vi "Main Tclk.vi"() -> ()   [LabVIEW 2018] (continued)
                  frame False {
                    n1784 = local read "AlnX array tiled"() -> (w6252:sgl[][][])
                    n1785 = local read "AlnY array tiled"() -> (w6253:sgl[][][])
                    n1786 = local read "Auto Focus"() -> (w6257:bool)
                    n1787 = local read "Auto Stig"() -> (w6258:bool)
                    n1788 = Empty Array?(array=w6252) -> (empty?=w6251:bool)
                    n1789 = Empty Array?(array=w6253) -> (empty?=w6250:bool)
                    n1790 = local write "Aln Options"(enum16{"Defaut", "Aln X", "Aln Y"}."Defaut" ("Stig Options")) -> ()
                    n1791 = Not(x=w6257) -> (.not. x?=w6259:bool)
                    n1792 = Not(x=w6258) -> (.not. x?=w6260:bool)
                    n1793 = And(x=w6251, y=w6250) -> (x .and. y?=w6255:bool)
                    n1794 = Compound Arithmetic op=AND(w6255, w6259, w6260) -> (w6256:bool)
                    n1795 = case shown="False" w6255 {
                      frame False {
                        n1796 = property on="Auto Align" class="Bool (strict)"("DisabledEnum"=T44."Disabled and Grayed Out" ("Disabled")) -> ()  [unwired: 2 in, 2 out]
                      }
                      frame True {
                      }
                    }
                    n1797 = case shown="True" w6256 {
                      frame False {
                      }
                      frame True {
                        w6261 = T44."Enabled" ("Disabled")
                        n1798 = property on="Auto Focus" class="Bool (strict)"("DisabledEnum"=w6261) -> ()  [unwired: 2 in, 2 out]
                        n1799 = property on="Auto Stig" class="Bool (strict)"("DisabledEnum"=w6261) -> ()  [unwired: 2 in, 2 out]
                      }
                    }
                  }
                  frame True {
                    w6265 = T44."Disabled and Grayed Out" ("Disabled")
                    n1800 = local read "SEM Scan Parameters"() -> (w6269:T26)
                    n1801 = local read "AA Count"() -> (w6264:u8)
                    n1802 = local read "Aln Options"() -> (w6273:enum16{"Defaut", "Aln X", "Aln Y"})
                    n1803 = Increment(x=w6264) -> (x+1=w6270:u8)
                    n1804 = Equal To 0?(x=w6264) -> (x = 0?=w6263:bool)
                    n1805 = local write "AA Count"(w6270) -> ()
                    n1806 = Unbundle By Name(w6269) -> ("Y tiles"=w6268:u8, "X tiles"=w6267:u8)
                    n1807 = Equal?(x=w6273, y=enum16{"Defaut", "Aln X", "Aln Y"}."Defaut" ("Aln Options")) -> (x = y?=w6271:bool)
                    n1808 = property on="Auto Focus" class="Bool (strict)"("DisabledEnum"=w6265) -> ()  [unwired: 2 in, 2 out]
                    n1809 = And(x=w6263, y=w6271) -> (x .and. y?=w6272:bool)
                    n1810 = case shown="True" w6272 {
                      tunnel: w6268 -> [_ w6277]
                      tunnel: w6267 -> [_ w6276]
                      frame False {
                      }
                      frame True {
                        n1811 = Initialize Array(FALSE ("ASX Success"), w6277, w6276) -> (w6280:bool[][])
                        n1812 = Initialize Array(u8 0 ("Skip Steps"), w6277, w6276) -> (w6275:u8[][])
                        n1813 = local write "AAX Success tiled"(w6280) -> ()
                        n1814 = local write "AAY Success tiled"(w6280) -> ()
                        n1815 = local write "Skip Steps tiled"(w6275) -> ()
                        n1816 = local write "Aln Options"(enum16{"Defaut", "Aln X", "Aln Y"}."Aln X" ("Stig Options")) -> ()
                        n1817 = local write "Image Tabs"(T37."Auto Focus / Stig / Align" ("Image Tabs")) -> ()
                      }
                    }
                    n1818 = property on="Auto Stig" class="Bool (strict)"("DisabledEnum"=w6265) -> ()  [unwired: 2 in, 2 out]
                  }
                }
              }
              frame #16 {
                n1819 = local read "SEM Scan Parameters"() -> (w6319:T26)
                n1820 = local read "FIB slice #"() -> (w6329:u32)
                n1821 = local read "Machine Type"() -> (w6316:u8)
                n1822 = shared-variable "My Computer\\Zeiss Library.lvlib\\FIB Slice #"(w6329) -> ()  [unwired: 1 in, 1 out]
                n1823 = Equal To 0?(x=w6329) -> (x = 0?=w6352:bool)
                n1824 = Or(x=w6352, y="Reset Focus") -> (x .or. y?=w6321:bool)
                n1825 = local read "Milling para"() -> (w6345:T35)
                n1826 = local read "FIB-SEM Angle"() -> (w6348:dbl)
                n1827 = case shown="False" w6321 {
                  tunnel: [w6358 w6365] -> w6325
                  tunnel: [w6357 w6364] -> w6324
                  tunnel: [w6356 w6363] -> w6326
                  tunnel: [w6355 w6362] -> w6323
                  tunnel: [w6354 w6361] -> w6322
                  tunnel: w6319 -> [w6353 w6360]
                  tunnel: w6316 -> [_ w6359]
                  frame False {
                    n1828 = Unbundle By Name(w6353) -> ("WD (mm)"=w6356:sgl[][], "X stig"=w6358:sgl[][], "Y stig"=w6357:sgl[][], "X aln"=w6355:sgl[][], "Y aln"=w6354:sgl[][])
                  }
                  frame True {
                    n1829 = stacked-sequence {
                      tunnel: [_ w6373] -> w6365
                      tunnel: [_ w6372] -> w6364
                      tunnel: [_ w6371] -> w6363
                      tunnel: [_ w6370] -> w6362
                      tunnel: [_ w6369] -> w6361
                      tunnel: w6360 -> [_ w6368]
                      tunnel: w6359 -> [_ w6367]
                      frame #0 {
                        n1830 = local read "SEM Options"() -> (→"Initial Options":T27)
                      }
                      frame #1 {
                        n1831 = case shown="2" w6367 {
                          tunnel: [w6381 w6460] -> w6373
                          tunnel: [w6380 w6459] -> w6372
                          tunnel: [w6379 w6461] -> w6371
                          tunnel: [w6378 w6458] -> w6370
                          tunnel: [w6377 w6457] -> w6369
                          tunnel: w6368 -> [w6374 _]
                          frame 0, Default {
                            n1832 = local read "Hardware Configuration"() -> (w6376:T25)
                            n1833 = Unbundle By Name(w6376) -> ("Eanable COM"=w6375:bool)
                            n1834 = case shown="True" w6375 {
                              tunnel: [w6385 w6395] -> w6381
                              tunnel: [w6384 w6394] -> w6380
                              tunnel: [w6386 w6400] -> w6379
                              tunnel: [w6383 w6393] -> w6378
                              tunnel: [w6382 w6392] -> w6377
                              tunnel: w6374 -> [w6387 _]
                              frame False {
                                n1835 = Unbundle By Name(w6387) -> ("WD (mm)"=w6386:sgl[][], "X stig"=w6385:sgl[][], "Y stig"=w6384:sgl[][], "X aln"=w6383:sgl[][], "Y aln"=w6382:sgl[][])
                              }
                              frame True {
                                w6414 = TRUE ("Initialization")
                                w6405 = 0 ("offset past token")
                                n1836 = local read "COM port"() -> (w6418:refnum<visa-resource-name>)
                                n1837 = call "Remcon32 command.vi"("Initialization"=w6414, "SEM command"="sti? " ("write buffer"), "COM port in"=w6418) -> ("error out"=w6408:errorcluster, "SEM reply"=w6415:string, "COM port out"=w6410:refnum<visa-resource-name>)  [unwired: 2 in, 4 out]
                                n1838 = while {
                                shift-right: [w6436] -> _
                                shift-left: w6405 -> [w6439]
                                tunnel: [w6437] -> w6421 mode=indexing
                                tunnel: w6415 -> [w6434]
                                stop <- w6435 stop-if-true
                                n1839 = Scan String For Tokens(8:w6439, 9:w6434) -> (1:w6437:string, 2:w6436:i32)  [unwired: 1 in, 5 out]
                                n1840 = Less?(x=w6436, y=0) -> (x < y?=w6435:bool)
                                }
                                n1841 = call "Remcon32 command.vi"("error in"=w6408, "SEM command"="aln? " ("write buffer"), "COM port in"=w6410) -> ("error out"=w6407:errorcluster, "SEM reply"=w6406:string, "COM port out"=w6409:refnum<visa-resource-name>)  [unwired: 2 in, 4 out]
                                n1842 = while {
                                shift-right: [w6427] -> _
                                shift-left: w6405 -> [w6430]
                                tunnel: [w6428] -> w6411 mode=indexing
                                tunnel: w6406 -> [w6425]
                                stop <- w6426 stop-if-true
                                n1843 = Scan String For Tokens(8:w6430, 9:w6425) -> (1:w6428:string, 2:w6427:i32)  [unwired: 1 in, 5 out]
                                n1844 = Less?(x=w6427, y=0) -> (x < y?=w6426:bool)
                                }
                                n1845 = for {
                                tunnel: w6421 -> [w6433] mode=indexing
                                tunnel: [w6432] -> w6420 mode=indexing
                                n1846 = Fract/Exp String To Number(string=w6433, default (0 dbl)=sgl 0.0 ("default (0 DBL)")) -> (number=w6432:sgl)  [unwired: 3 out]
                                }
                                n1847 = for {
                                tunnel: w6411 -> [w6424] mode=indexing
                                tunnel: [w6423] -> w6412 mode=indexing
                                n1848 = Fract/Exp String To Number(string=w6424, default (0 dbl)=sgl 0.0 ("default (0 DBL)")) -> (number=w6423:sgl)  [unwired: 3 out]
                                }
                                n1849 = call "Remcon32 command.vi"("Close session"=w6414, "error in"=w6407, "SEM command"="foc? " ("write buffer"), "COM port in"=w6409) -> ("SEM reply"=w6416:string)  [unwired: 1 in, 6 out]
                                n1850 = local read "WD Stig Aln tile offsets"() -> (w6403:T3)
                                n1851 = Fract/Exp String To Number(string=w6416, default (0 dbl)=sgl 0.0 ("default (0 DBL)")) -> (number=w6401:sgl)  [unwired: 3 out]
                                n1852 = Index Array(array=w6420) -> (element #1=w6391:sgl, element #2=w6390:sgl)  [unwired: 2 in]
                                n1853 = Index Array(array=w6412) -> (element #1=w6389:sgl, element #2=w6388:sgl)  [unwired: 2 in]
                                n1854 = Unbundle By Name(w6403) -> ("dWD"=w6402:sgl[][], "dX stig"=w6399:sgl[][], "dY stig"=w6398:sgl[][], "dX aln"=w6397:sgl[][], "dY aln"=w6396:sgl[][])
                                n1855 = Add(x=w6402, y=w6401) -> (x+y=w6400:sgl[][])
                                n1856 = Add(x=w6399, y=w6391) -> (x+y=w6395:sgl[][])
                                n1857 = Add(x=w6398, y=w6390) -> (x+y=w6394:sgl[][])
                                n1858 = Add(x=w6397, y=w6389) -> (x+y=w6393:sgl[][])
                                n1859 = Add(x=w6396, y=w6388) -> (x+y=w6392:sgl[][])
                              }
                            }
                          }
                          frame 2 {
                            n1860 = local read "Api"() -> (w6452:refnum<k7>)
                            n1861 = call "SmartSEM Remote API get float.vi"("lpszParam"="AP_WD", "Api"=w6452) -> ("error out"=w6441:errorcluster, "vValue"=w6454:sgl)  [unwired: 7 in, 1 out]
                            n1862 = call "SmartSEM Remote API get float.vi"("error in"=w6441, "lpszParam"="AP_STIG_X", "Api"=w6452) -> ("error out"=w6440:errorcluster, "vValue"=w6447:sgl, "Api out"=w6450:refnum<k7>)  [unwired: 6 in]
                            n1863 = call "SmartSEM Remote API get float.vi"("error in"=w6440, "lpszParam"="AP_STIG_Y", "Api"=w6452) -> ("error out"=w6445:errorcluster, "vValue"=w6442:sgl, "Api out"=w6446:refnum<k7>)  [unwired: 6 in]
                            n1864 = expression code="x*1000"(w6454) -> (w6456:sgl)
                            n1865 = call "SmartSEM Remote API get float.vi"("error in"=w6440, "lpszParam"="AP_APERTURE_ALIGN_X", "Api"=w6450) -> ("vValue"=w6448:sgl)  [unwired: 6 in, 2 out]
                            n1866 = call "SmartSEM Remote API get float.vi"("error in"=w6445, "lpszParam"="AP_APERTURE_ALIGN_Y", "Api"=w6446) -> ("vValue"=w6443:sgl)  [unwired: 6 in, 2 out]
                            n1867 = local read "WD Stig Aln tile offsets"() -> (w6462:T3)
                            n1868 = Unbundle By Name(w6462) -> ("dWD"=w6463:sgl[][], "dX stig"=w6464:sgl[][], "dY stig"=w6465:sgl[][], "dX aln"=w6466:sgl[][], "dY aln"=w6467:sgl[][])
                            n1869 = Add(x=w6463, y=w6456) -> (x+y=w6461:sgl[][])
                            n1870 = Add(x=w6464, y=w6447) -> (x+y=w6460:sgl[][])
                            n1871 = Add(x=w6465, y=w6442) -> (x+y=w6459:sgl[][])
                            n1872 = Add(x=w6466, y=w6448) -> (x+y=w6458:sgl[][])
                            n1873 = Add(x=w6467, y=w6443) -> (x+y=w6457:sgl[][])
                          }
                        }
                      }
                    }
                  }
                }
                n1874 = Unbundle By Name(w6319) -> ("X center (um)"=w6318:sgl, "Y center (um)"=w6317:sgl)
                n1875 = Unbundle By Name(w6345) -> ("Z-step (nm)"=w6315:dbl, "Lines auto pause"=w6314:u16)
                n1876 = expression code="cos(x/180*pi)"(w6348) -> (w6349:dbl)
                n1877 = local read "SEM FOV"() -> (w6336:dbl)
                n1878 = Unbundle By Name(w6319) -> ("X size (um)"=w6328:sgl, "Y size (um)"=w6327:sgl)
                n1879 = Compound Arithmetic op=MULTIPLY(w6315, w6314, w6349) -> (w6344:dbl)
                n1880 = Subtract(x=w6344, y="Y shift (nm/image)") -> (x-y=w6338:dbl)
                n1881 = expression code="x/1000"(w6338) -> (w6337:dbl)
                n1882 = expression code="x/1000"("X shift (nm/image)") -> (w6339:sgl)
                n1883 = Subtract(x=w6336, y=w6328) -> (x-y=w6335:dbl)
                n1884 = Subtract(x=w6336, y=w6327) -> (x-y=w6332:dbl)
                n1885 = Subtract(x=w6317, y=w6337) -> (x-y=w6347:dbl)
                n1886 = expression code="x/2"(w6335) -> (w6334:dbl)
                n1887 = expression code="x/2"(w6332) -> (w6331:dbl)
                n1888 = Add(x=w6318, y=w6339) -> (x+y=w6342:sgl)
                n1889 = Negate(x=w6334) -> (-x=w6333:dbl)
                n1890 = Negate(x=w6331) -> (-x=w6330:dbl)
                n1891 = In Range and Coerce(upper limit=w6334, x=w6342, lower limit=w6333) -> (coerced(x)=w6341:dbl)  [unwired: 1 out]
                n1892 = In Range and Coerce(upper limit=w6331, x=w6347, lower limit=w6330) -> (coerced(x)=w6346:dbl)  [unwired: 1 out]
                n1893 = local read "SEM Scan Parameters"() -> (w6351:T26)
                n1894 = Bundle By Name(cluster=w6351, "WD (mm)"=w6326, "X stig"=w6325, "Y stig"=w6324, "X aln"=w6323, "Y aln"=w6322, "X center (um)"=w6341, "Y center (um)"=w6346) -> (w6350:T26)
                n1895 = local write "SEM Scan Parameters"(w6350) -> ()
              }
              frame #17 {
                n1896 = local read "SEM Scan Parameters"() -> (w6472:T26)
                n1897 = local read "AF Count"() -> (w6468:u8)
                n1898 = local read "Auto Focus"() -> (w6474:bool)
                n1899 = Unbundle By Name(w6472) -> ("WD (mm)"=w6473:sgl[][])
                n1900 = case shown="False" w6474 {
                  tunnel: w6473 -> [w6482 w6492]
                  tunnel: [w6479 w6487] -> w6471
                  tunnel: [sgl[][][] [] ("Array") w6488] -> w6469
                  tunnel: w6468 -> [_ w6489]
                  frame False {
                    n1901 = local read "Milling para"() -> (w6484:T35)
                    n1902 = To Double Precision Float(number=w6482) -> (double precision float=w6478:dbl[][])
                    n1903 = Unbundle By Name(w6484) -> ("Z-step (nm)"=w6477:dbl, "Lines auto pause"=w6475:u16)
                    n1904 = expression code="1/sin(x/180*pi)"("FIB-SEM Angle") -> (w6483:dbl)
                    n1905 = expression code="x/1e6"(w6477) -> (w6476:dbl)
                    n1906 = Compound Arithmetic op=MULTIPLY(w6476, w6475, w6483) -> (w6486:dbl)
                    n1907 = Add(x=w6478, y=w6486) -> (x+y=w6481:dbl[][])
                    n1908 = To Single Precision Float(number=w6481) -> (single precision float=w6479:sgl[][])
                  }
                  frame True {
                    n1909 = property on="AF Steps" class="DigNum (strict)"("DisabledEnum"=T44."Disabled and Grayed Out" ("Disabled")) -> ()  [unwired: 2 in, 2 out]
                    n1910 = for {
                      tunnel: w6489 -> [w6498]
                      tunnel: w6492 -> [w6497] mode=indexing
                      tunnel: [w6496] -> w6491 mode=indexing
                      tunnel: [w6495] -> w6490 mode=indexing
                      i -> [w6494]
                      n1911 = for {
                        tunnel: w6498 -> [w6503]
                        tunnel: w6497 -> [w6506] mode=indexing
                        tunnel: [w6505] -> w6496 mode=indexing
                        tunnel: [w6504] -> w6495 mode=indexing
                        tunnel: w6494 -> [w6501]
                        i -> [w6499]
                        n1912 = Decrement(x=w6503) -> (x-1=w6500:u8)
                        n1913 = Equal To 0?(x=w6500) -> (x = 0?=w6502:bool)
                        n1914 = case shown="False" w6502 {
                          tunnel: [w6510 w6514] -> w6507
                          tunnel: w6506 -> [_ w6515]
                          tunnel: [w6510 w6514] -> w6504
                          tunnel: w6501 -> [w6509 _]
                          tunnel: w6499 -> [w6508 _]
                          frame False {
                            n1915 = local read "WD array tiled"() -> (w6511:sgl[][][])
                            n1916 = Index Array(array=w6511, index (dim 0)=w6509, index (dim 1)=w6508) -> (element=w6510:sgl[])  [unwired: 1 in]
                          }
                          frame True {
                            n1917 = local read "AF Range (nm)"() -> (w6513:sgl)
                            n1918 = local read "AF Steps"() -> (w6512:u8)
                            n1919 = expression code="x/1e6"(w6513) -> (w6516:sgl)
                            n1920 = call "Step down array.vi"("Steps"=w6512, "Range"=w6516, "Center"=w6515) -> ("Array"=w6514:dbl[])  [unwired: 8 in]
                          }
                        }
                        n1921 = Index Array(array=w6507, index=w6500) -> (element=w6505:dbl)
                      }
                    }
                    n1922 = To Single Precision Float(number=w6490) -> (single precision float=w6488:sgl[][][])
                    n1923 = To Single Precision Float(number=w6491) -> (single precision float=w6487:sgl[][])
                  }
                }
                n1924 = Bundle By Name(cluster=w6472, "WD (mm)"=w6471) -> (w6470:T26)
                n1925 = local write "WD array tiled"(w6469) -> ()
                n1926 = local write "SEM Scan Parameters"(w6470) -> ()
              }
              frame #18 {
                n1927 = local read "SEM Scan Parameters"() -> (w6524:T26)
                n1928 = local read "AS Count"() -> (w6518:u8)
                n1929 = local read "AA Count"() -> (w6517:u8)
                n1930 = Unbundle By Name(w6524) -> ("X stig"=w6527:sgl[][], "Y stig"=w6528:sgl[][])
                n1931 = Unbundle By Name(w6524) -> ("X aln"=w6530:sgl[][], "Y aln"=w6531:sgl[][])
                n1932 = case shown="\"Stig X\"" "Stig Options" {
                  tunnel: [w6598 w6605 w6631] -> w6523
                  tunnel: [w6597 w6602 w6633] -> w6522
                  tunnel: w6527 -> [w6598 w6603 w6631]
                  tunnel: w6528 -> [w6597 w6602 w6632]
                  tunnel: [w6596 w6601 dbl[][][] [] ("Array")] -> w6529
                  tunnel: [w6596 dbl[][][] [] ("Array") w6630] -> w6532
                  tunnel: w6518 -> [_ w6600 w6629]
                  frame "Defaut", Default {
                    w6596 = dbl[][][] [] ("Array")
                  }
                  frame "Stig X" {
                    n1933 = property on="AS Steps" class="DigNum (strict)"("DisabledEnum"=T44."Disabled and Grayed Out" ("Disabled")) -> ()  [unwired: 2 in, 2 out]
                    n1934 = for {
                      tunnel: w6600 -> [w6610]
                      tunnel: [w6609] -> w6605 mode=indexing
                      tunnel: w6603 -> [w6608] mode=indexing
                      tunnel: [w6607] -> w6601 mode=indexing
                      i -> [w6606]
                      n1935 = for {
                        tunnel: w6610 -> [w6615]
                        tunnel: [w6618] -> w6609 mode=indexing
                        tunnel: w6608 -> [w6617] mode=indexing
                        tunnel: [w6616] -> w6607 mode=indexing
                        tunnel: w6606 -> [w6612]
                        i -> [w6611]
                        n1936 = Decrement(x=w6615) -> (x-1=w6613:u8)
                        n1937 = Equal To 0?(x=w6613) -> (x = 0?=w6614:bool)
                        n1938 = case shown="False" w6614 {
                          tunnel: [w6620 w6626] -> w6619
                          tunnel: w6617 -> [_ w6627]
                          tunnel: [w6620 w6626] -> w6616
                          tunnel: w6612 -> [w6622 _]
                          tunnel: w6611 -> [w6621 _]
                          frame False {
                            n1939 = local read "StigX array tiled"() -> (w6623:sgl[][][])
                            n1940 = Index Array(array=w6623, index (dim 0)=w6622, index (dim 1)=w6621) -> (element=w6620:sgl[])  [unwired: 1 in]
                          }
                          frame True {
                            n1941 = local read "AS Range (%)"() -> (w6625:sgl)
                            n1942 = local read "AS Steps"() -> (w6624:u8)
                            n1943 = call "Step down array.vi"("Steps"=w6624, "Range"=w6625, "Center"=w6627) -> ("Array"=w6626:dbl[])  [unwired: 8 in]
                          }
                        }
                        n1944 = Index Array(array=w6619, index=w6613) -> (element=w6618:dbl)
                      }
                    }
                  }
                  frame "Stig Y" {
                    n1945 = property on="AS Steps" class="DigNum (strict)"("DisabledEnum"=T44."Disabled and Grayed Out" ("Disabled")) -> ()  [unwired: 2 in, 2 out]
                    n1946 = for {
                      tunnel: w6629 -> [w6639]
                      tunnel: [w6638] -> w6633 mode=indexing
                      tunnel: [w6637] -> w6630 mode=indexing
                      tunnel: w6632 -> [w6636] mode=indexing
                      i -> [w6635]
                      n1947 = for {
                        tunnel: w6639 -> [w6643]
                        tunnel: [w6647] -> w6638 mode=indexing
                        tunnel: [w6646] -> w6637 mode=indexing
                        tunnel: w6636 -> [w6645] mode=indexing
                        tunnel: w6635 -> [w6641]
                        i -> [w6640]
                        n1948 = Decrement(x=w6643) -> (x-1=w6642:u8)
                        n1949 = Equal To 0?(x=w6642) -> (x = 0?=w6644:bool)
                        n1950 = case shown="False" w6644 {
                          tunnel: [w6649 w6654] -> w6648
                          tunnel: [w6649 w6654] -> w6646
                          tunnel: w6645 -> [_ w6653]
                          tunnel: w6641 -> [w6651 _]
                          tunnel: w6640 -> [w6650 _]
                          frame False {
                            n1951 = local read "StigY array tiled"() -> (w6652:sgl[][][])
                            n1952 = Index Array(array=w6652, index (dim 0)=w6651, index (dim 1)=w6650) -> (element=w6649:sgl[])  [unwired: 1 in]
                          }
                          frame True {
                            n1953 = local read "AS Range (%)"() -> (w6655:sgl)
                            n1954 = local read "AS Steps"() -> (w6656:u8)
                            n1955 = call "Step down array.vi"("Steps"=w6656, "Range"=w6655, "Center"=w6653) -> ("Array"=w6654:dbl[])  [unwired: 8 in]
                          }
                        }
                        n1956 = Index Array(array=w6648, index=w6642) -> (element=w6647:dbl)
                      }
                    }
                  }
                }
                n1957 = case shown="\"Aln Y\"" "Aln Options" {
                  tunnel: [w6537 w6544 w6572] -> w6521
                  tunnel: [w6536 w6540 w6570] -> w6520
                  tunnel: w6530 -> [w6537 w6542 w6572]
                  tunnel: w6531 -> [w6536 w6540 w6571]
                  tunnel: [w6535 w6541 dbl[][][] [] ("Array")] -> w6533
                  tunnel: [w6535 dbl[][][] [] ("Array") w6569] -> w6534
                  tunnel: w6517 -> [_ w6539 w6568]
                  frame "Defaut", Default {
                    w6535 = dbl[][][] [] ("Array")
                  }
                  frame "Aln X" {
                    n1958 = property on="AA Steps" class="DigNum (strict)"("DisabledEnum"=T44."Disabled and Grayed Out" ("Disabled")) -> ()  [unwired: 2 in, 2 out]
                    n1959 = for {
                      tunnel: [w6549] -> w6544 mode=indexing
                      tunnel: w6542 -> [w6548] mode=indexing
                      tunnel: [w6547] -> w6541 mode=indexing
                      tunnel: w6539 -> [w6546]
                      i -> [w6545]
                      n1960 = for {
                        tunnel: [w6557] -> w6549 mode=indexing
                        tunnel: w6548 -> [w6556] mode=indexing
                        tunnel: [w6555] -> w6547 mode=indexing
                        tunnel: w6546 -> [w6554]
                        tunnel: w6545 -> [w6551]
                        i -> [w6550]
                        n1961 = Decrement(x=w6554) -> (x-1=w6552:u8)
                        n1962 = Equal To 0?(x=w6552) -> (x = 0?=w6553:bool)
                        n1963 = case shown="False" w6553 {
                          tunnel: [w6559 w6565] -> w6558
                          tunnel: w6556 -> [_ w6566]
                          tunnel: [w6559 w6565] -> w6555
                          tunnel: w6551 -> [w6560 _]
                          tunnel: w6550 -> [w6561 _]
                          frame False {
                            n1964 = local read "AlnX array tiled"() -> (w6562:sgl[][][])
                            n1965 = Index Array(array=w6562, index (dim 0)=w6560, index (dim 1)=w6561) -> (element=w6559:sgl[])  [unwired: 1 in]
                          }
                          frame True {
                            n1966 = local read "AA Range (%)"() -> (w6563:sgl)
                            n1967 = local read "AA Steps"() -> (w6564:u8)
                            n1968 = call "Step down array.vi"("Steps"=w6564, "Range"=w6563, "Center"=w6566) -> ("Array"=w6565:dbl[])  [unwired: 8 in]
                          }
                        }
                        n1969 = Index Array(array=w6558, index=w6552) -> (element=w6557:dbl)
                      }
                    }
                  }
                  frame "Aln Y" {
                    n1970 = property on="AA Steps" class="DigNum (strict)"("DisabledEnum"=T44."Disabled and Grayed Out" ("Disabled")) -> ()  [unwired: 2 in, 2 out]
                    n1971 = for {
                      tunnel: w6568 -> [w6578]
                      tunnel: w6571 -> [w6577] mode=indexing
                      tunnel: [w6576] -> w6570 mode=indexing
                      tunnel: [w6575] -> w6569 mode=indexing
                      i -> [w6574]
                      n1972 = for {
                        tunnel: w6578 -> [w6583]
                        tunnel: w6577 -> [w6586] mode=indexing
                        tunnel: [w6585] -> w6576 mode=indexing
                        tunnel: [w6584] -> w6575 mode=indexing
                        tunnel: w6574 -> [w6580]
                        i -> [w6579]
                        n1973 = Decrement(x=w6583) -> (x-1=w6582:u8)
                        n1974 = Equal To 0?(x=w6582) -> (x = 0?=w6581:bool)
                        n1975 = case shown="False" w6581 {
                          tunnel: [w6588 w6592] -> w6587
                          tunnel: w6586 -> [_ w6593]
                          tunnel: [w6588 w6592] -> w6584
                          tunnel: w6580 -> [w6589 _]
                          tunnel: w6579 -> [w6590 _]
                          frame False {
                            n1976 = local read "AlnY array tiled"() -> (w6591:sgl[][][])
                            n1977 = Index Array(array=w6591, index (dim 0)=w6589, index (dim 1)=w6590) -> (element=w6588:sgl[])  [unwired: 1 in]
                          }
                          frame True {
                            n1978 = local read "AA Steps"() -> (w6595:u8)
                            n1979 = local read "AA Range (%)"() -> (w6594:sgl)
                            n1980 = call "Step down array.vi"("Steps"=w6595, "Range"=w6594, "Center"=w6593) -> ("Array"=w6592:dbl[])  [unwired: 8 in]
                          }
                        }
                        n1981 = Index Array(array=w6587, index=w6582) -> (element=w6585:dbl)
                      }
                    }
                  }
                }
                n1982 = local write "StigX array tiled"(w6529) -> ()
                n1983 = local write "StigY array tiled"(w6532) -> ()
                n1984 = local write "AlnX array tiled"(w6533) -> ()
                n1985 = local write "AlnY array tiled"(w6534) -> ()
                n1986 = Bundle By Name(cluster=w6524, "X stig"=w6523, "Y stig"=w6522, "X aln"=w6521, "Y aln"=w6520) -> (w6519:T26)
                n1987 = local write "SEM Scan Parameters"(w6519) -> ()
              }
              frame #19 {
                n1988 = local read "Tiled scan inputs"() -> (w6659:T6)
                n1989 = local read "SEM HW Config"() -> (w6660:T9)
                n1990 = local read "Detector Information"() -> (w6661:T8)
                n1991 = local read "SEM Scan Parameters"() -> (w6662:T26)
                n1992 = local read "SEM Options"() -> (w6663:T27)
                n1993 = local read "Focus Index Options"() -> (w6657:T28)
                n1994 = local read "File Information"() -> (w6664:T31)
                n1995 = local read "Milling para"() -> (w6665:T35)
                n1996 = Bundle By Name(cluster=w6659, "HW Config"=w6660, "Det Info"=w6661, "SEM Scan Parameters"=w6662, "SEM Options"=w6663, "Focus Index Options"=w6657, "File Information"=w6664, "Milling para"=w6665) -> (w6658:T6)
                n1997 = local write "Tiled scan inputs"(w6658) -> ()
              }
              frame #20 {
                n1998 = local read "FIB"() -> (w6668:bool)
                n1999 = local read "Stop"() -> (w6669:bool)
                n2000 = Not(x=w6669) -> (.not. x?=w6667:bool)
                n2001 = And(x=w6668, y=w6667) -> (x .and. y?=w6666:bool)
                n2002 = case shown="True" w6666 {
                  frame False {
                  }
                  frame True {
                    w6715 = TRUE ("SEM Options.Set WD")
                    w6679 = 10.0 ("rate")
                    n2003 = local read "Tiled scan inputs"() -> (w6720:T6)
                    n2004 = Bundle By Name(cluster=w6720, "SEM Options.Set WD"=w6715, "SEM Options.Set stig"=w6715, "SEM Options.Set aln"=w6715, "SEM Options.Freeze"=w6715) -> (w6719:T6)
                    n2005 = call "2D scan tiled.vi"("Tiled scan inputs"=w6719) -> ("Image Focus Index Tiled"=w6714:T52, "Image Focus Index Array Tiled"=w6713:T53, "Low res scale Tiled (um/pix)"=→"Low res scale tiled":dbl[][], "Single scan outputs"=w6718:T54, "SEM Spec. I Tiled (nA)"=w6691:sgl[][], "8-bit over scale"=w6703:bool[])  [unwired: 5 in]
                    n2006 = Array Size(array=w6691) -> (size(s)=w6692:i32[])
                    n2007 = local read "FI Detector"() -> (w6732:u16)
                    n2008 = local read "SEM Status"() -> (w6741:T12)
                    n2009 = Unbundle By Name(w6741) -> ("Scan time (m)"=w6746:dbl, "Scan time (s)"=w6676:dbl)
                    n2010 = Multiply Array Elements(1:w6692) -> (0:w6693:i32)
                    n2011 = Reshape Array(w6691, w6693) -> (w6694:sgl[])
                    n2012 = Unbundle By Name(w6718) -> ("SEM Parameters"=w6717:T13, "Image Focus Index"=w6709:T14, "FIB parameters"=→"FIB Parameters":T56)
                    n2013 = case shown="0, Default" w6732 {
                      tunnel: w6714 -> [w6764 w6768 w6772 w6776]
                      tunnel: [w6763 w6765 w6771 w6775] -> w6748
                      tunnel: w6713 -> [w6762 w6767 w6770 w6774]
                      tunnel: [w6761 w6766 w6769 w6773] -> w6747
                      frame 0, Default {
                        n2014 = Unbundle By Name(w6764) -> ("A Img Focus Index"=w6763:sgl[][])
                        n2015 = Unbundle By Name(w6762) -> ("A Img Focus Index array"=w6761:sgl[][][][])
                      }
                      frame 1 {
                        n2016 = Unbundle By Name(w6768) -> ("B Img Focus Index"=w6765:sgl[][])
                        n2017 = Unbundle By Name(w6767) -> ("B Img Focus Index array"=w6766:sgl[][][][])
                      }
                      frame 2 {
                        n2018 = Unbundle By Name(w6772) -> ("C Img Focus Index"=w6771:sgl[][])
                        n2019 = Unbundle By Name(w6770) -> ("C Img Focus Index array"=w6769:sgl[][][][])
                      }
                      frame 3 {
                        n2020 = Unbundle By Name(w6776) -> ("D Img Focus Index"=w6775:sgl[][])
                        n2021 = Unbundle By Name(w6774) -> ("D Img Focus Index array"=w6773:sgl[][][][])
                      }
                    }
                    "Focus Index tiled" <- w6748
                    "Focus Index array tiled" <- w6747
                    n2022 = call-poly <vilib>:"Mean.vi"("X"=w6694) -> ("mean"=→"SEM Specimen I":dbl)  [unwired: 1 out]
                    n2023 = Multiply(x=60.0, y=w6746) -> (x*y=w6744:dbl)
                    n2024 = local read "Pause for reheat"() -> (w6672:bool)
                    n2025 = Add(x=w6744, y=w6676) -> (x+y=w6682:dbl)
                    n2026 = In Range and Coerce(upper limit=60.0, x=w6682, lower limit=2.0) -> (coerced(x)=w6729:dbl)  [unwired: 1 out]
                    n2027 = local write "SEM Parameters"(w6717) -> ()
                    n2028 = local write "Image Focus Index"(w6709) -> ()
                    n2029 = Multiply(x=w6729, y=w6679) -> (x*y=w6675:dbl)
                    n2030 = Index Array(array=w6703, index #1=0 ("index"), index #2=1 ("index")) -> (element #1=w6706:bool, element #2=w6707:bool)
                    n2031 = Select(t="Pausing for FIB reheat ..." ("Status message"), s=w6672, f="SEM between FIB" ("Status message")) -> (s? t:f=w6671:string)
                    n2032 = for {
                      N: w6675 -> [_]
                      shift-right: [w6760] -> w6681
                      shift-left: sgl[][] [] -> [w6759]
                      tunnel: w6679 -> [w6757]
                      n2033 = shared-variable ".\\Zeiss Library.lvlib\\Logs"() -> (w6756:sgl[])  [unwired: 1 in, 1 out]
                      n2034 = expression code="1000/x"(w6757) -> (w6758:dbl)
                      n2035 = Wait Until Next ms Multiple(millisecond multiple=w6758) -> ()  [unwired: 1 out]
                      n2036 = Build Array (concatenate)(w6759, w6756) -> (w6760:sgl[][])
                    }
                    n2037 = local write "Det A over scale"(w6706) -> ()
                    n2038 = local write "Det B over scale"(w6707) -> ()
                    n2039 = Array Size(array=w6748) -> (size(s)=w6712:i32[])
                    n2040 = local write "Status message"(w6671) -> ()
                    n2041 = Multiply Array Elements(1:w6712) -> (0:w6711:i32)
                    n2042 = Reshape Array(w6748, w6711) -> (w6710:sgl[])
                    n2043 = call-poly <vilib>:"Mean.vi"("X"=w6710) -> ("mean"=→"Focus Index":dbl)  [unwired: 1 out]
                    n2044 = Delete From Array(array=w6681, length=15.0 ("rate"), index (row)=0 ("disabled index (col)")) -> (array with subset deleted=w6680:sgl[][])  [unwired: 1 in, 1 out]
                    n2045 = Transpose 2D Array(2D array=w6680) -> (transposed array=w6730:sgl[][])
                    n2046 = shared-variable ".\\Zeiss Library.lvlib\\Faraday cup offset"() -> (w6696:sgl)  [unwired: 1 in, 1 out]
                    n2047 = for {
                      tunnel: [w6755] -> w6723 mode=indexing
                      tunnel: w6730 -> [w6754] mode=indexing
                      n2048 = call-poly <vilib>:"Basic Averaged DC-RMS.vi"("signal in"=w6754) -> ("DC value"=w6755:dbl)  [unwired: 7 in, 3 out]
                    }
                    n2049 = local read "Alert Settings"() -> (w6689:T36)
                    n2050 = To Single Precision Float(number=w6723) -> (single precision float=w6733:sgl[])
                    n2051 = Unbundle By Name(w6689) -> ("Low limit (F)"=w6683:sgl, "High limit (F)"=w6684:sgl)
                    n2052 = Index Array(array=w6733) -> (element=w6677:sgl)  [unwired: 1 in]
                    n2053 = local read "Machine Type"() -> (w6727:u8)
                    n2054 = Subtract(x=w6677, y=w6696) -> (x-y=w6726:sgl)
                    n2055 = local read "Faraday Cup array"() -> (w6740:sgl[])
                    n2056 = local read "Specimen I array"() -> (w6739:sgl[])
                    n2057 = local read "Specimen I (nA)"() -> (w6724:sgl)
                    n2058 = local read "Beam Dump 2 (nA)"() -> (w6702:sgl)
                    n2059 = local read "Milling I array"() -> (w6699:sgl[])
                    n2060 = local read "Milling I (nA)"() -> (w6697:sgl)
                    n2061 = local read "Temp low limit array"() -> (w6687:sgl[])
                    n2062 = local read "Temp high limit array"() -> (w6686:sgl[])
                    n2063 = local read "Beam Dump 1 array"() -> (w6738:sgl[])
                    n2064 = local read "Beam Dump 2 array"() -> (w6700:sgl[])
                    n2065 = local read "Beam Dump 1 (nA)"() -> (w6725:sgl)
                    n2066 = case shown="2" w6727 {
                      tunnel: w6726 -> [w6749 _ _]
                      tunnel: [w6749 w6752 w6753] -> w6722
                      tunnel: w6725 -> [_ w6751 _]
                      tunnel: w6724 -> [_ w6750 _]
                      tunnel: w6677 -> [_ _ w6753]
                      frame 0, Default {
                      }
                      frame 1 {
                        n2067 = Subtract(x=w6751, y=w6750) -> (x-y=w6752:sgl)
                      }
                      frame 2 {
                      }
                    }
                    "Faraday Cup (nA)" <- w6722
                    n2068 = local read "Temp array"() -> (w6737:sgl[])
                    n2069 = local read "Temp (F)"() -> (w6721:sgl)
                    n2070 = Build Array (concatenate)(w6739, w6724) -> (w6735:sgl[])
                    n2071 = shared-variable ".\\Zeiss Library.lvlib\\Temp (F)"(w6721) -> ()  [unwired: 1 in, 1 out]
                    n2072 = shared-variable ".\\Zeiss Library.lvlib\\Faraday Cup (nA)"(w6722) -> ()  [unwired: 1 in, 1 out]
                    n2073 = Build Array (concatenate)(w6740, w6722) -> (w6736:sgl[])
                    n2074 = Build Array (concatenate)(w6738, w6725) -> (w6734:sgl[])
                    n2075 = Build Array (concatenate)(w6700, w6702) -> (w6701:sgl[])
                    n2076 = Build Array (concatenate)(w6699, w6697) -> (w6698:sgl[])
                    n2077 = Build Array (concatenate)(w6737, w6721) -> (w6728:sgl[])
                    n2078 = Build Array (concatenate)(w6687, w6683) -> (w6688:sgl[])
                    n2079 = Build Array (concatenate)(w6686, w6684) -> (w6685:sgl[])
                    n2080 = local write "Faraday Cup array"(w6736) -> ()
                    n2081 = local write "Specimen I array"(w6735) -> ()
                    n2082 = local write "Milling I array"(w6698) -> ()
                    n2083 = local write "Beam Dump 1 array"(w6734) -> ()
                    n2084 = local write "Beam Dump 2 array"(w6701) -> ()
                    n2085 = local write "Temp array"(w6728) -> ()
                    n2086 = local write "Temp low limit array"(w6688) -> ()
                    n2087 = local write "Temp high limit array"(w6685) -> ()
                  }
                }
              }
              frame #21 {
                n2088 = local read "FI array for stop limit"() -> (w6811:sgl[])
                n2089 = local read "Focus Index"() -> (w6778:sgl)
                n2090 = local read "Alert Settings"() -> (w6800:T36)
                n2091 = Build Array (concatenate)(w6811, w6778) -> (w6801:sgl[])
                n2092 = Unbundle By Name(w6800) -> ("FI low limit auto"=w6809:bool)
                n2093 = Unbundle By Name(w6800) -> ("FI stop limit auto"=w6804:bool)
                n2094 = local read "Auto re-engage"() -> (w6803:bool)
                n2095 = local write "FI array for stop limit"(w6801) -> ()
                n2096 = Array Size(array=w6801) -> (size(s)=w6808:i32)
                n2097 = Greater Or Equal?(x=w6808, y=5 ("x")) -> (x >= y?=w6805:bool)
                n2098 = Or(x=w6804, y=w6803) -> (x .or. y?=w6802:bool)
                n2099 = And(x=w6805, y=w6809) -> (x .and. y?=w6810:bool)
                n2100 = And(x=w6805, y=w6802) -> (x .and. y?=w6806:bool)
                n2101 = local read "Focus index array"() -> (w6785:sgl[])
                n2102 = case shown="True" w6810 {
                  tunnel: w6800 -> [w6822 w6832]
                  tunnel: w6801 -> [_ w6828]
                  tunnel: [w6822 w6823] -> w6786
                  frame False {
                  }
                  frame True {
                    w6827 = 0.2 ("Minimum half range")
                    n2103 = call "Auto limits.vi"("lower band factor"=w6827, "upper band factor"=w6827, "Method"="sqrt of mean", "Minimum half range"=0.1, "Length"=5, "Input array"=w6828) -> ("Low limit"=w6826:dbl)  [unwired: 3 in, 2 out]
                    n2104 = Max & Min(x=w6826, y=0.0) -> (max(x,y)=w6830:dbl)  [unwired: 1 out]
                    n2105 = Bundle By Name(cluster=w6832, "Focus index low limit"=w6830) -> (w6823:T36)
                    n2106 = local write "Alert Settings"(w6823) -> ()
                  }
                }
                n2107 = case shown="True" w6806 {
                  tunnel: w6800 -> [_ w6820]
                  tunnel: w6801 -> [_ w6819]
                  frame False {
                  }
                  frame True {
                    w6813 = 0.4 ("Minimum half range")
                    n2108 = call "Auto limits.vi"("lower band factor"=w6813, "upper band factor"=w6813, "Method"="sqrt of mean", "Minimum half range"=0.4, "Length"=10, "Input array"=w6819) -> ("Low limit"=w6818:dbl)  [unwired: 3 in, 2 out]
                    n2109 = Max & Min(x=w6818, y=0.0) -> (max(x,y)=w6816:dbl)  [unwired: 1 out]
                    n2110 = Bundle By Name(cluster=w6820, "Focus index stop limit"=w6816) -> (w6821:T36)
                    n2111 = local write "Alert Settings"(w6821) -> ()
                  }
                }
                n2112 = Build Array (concatenate)(w6785, w6778) -> (w6779:sgl[])
                n2113 = local write "Focus index array"(w6779) -> ()
                n2114 = Unbundle By Name(w6786) -> ("Focus index low limit"=w6777:sgl)
                n2115 = local read "Auto Focus"() -> (w6797:bool)
                n2116 = local read "Auto Stig"() -> (w6798:bool)
                n2117 = local read "Auto Align"() -> (w6793:bool)
                n2118 = Divide(x="Smart upload FI threshold", y=100.0) -> (x/y=w6782:dbl)
                n2119 = Not(x=w6797) -> (.not. x?=w6792:bool)
                n2120 = Not(x=w6798) -> (.not. x?=w6791:bool)
                n2121 = Not(x=w6793) -> (.not. x?=w6790:bool)
                n2122 = Less Or Equal?(x=w6778, y=w6777) -> (x <= y?=w6794:bool)
                n2123 = Compound Arithmetic op=AND(w6792, w6791, w6790) -> (w6789:bool)
                n2124 = Multiply(x=w6777, y=w6782) -> (x*y=w6780:dbl)
                n2125 = Compound Arithmetic op=AND(w6794, w6789) -> (→"Focus index warning active":bool)
                n2126 = Greater Or Equal?(x=w6780, y=w6778) -> (x >= y?=→"Smart upload fail":bool)
                n2127 = local read "FI low limit array"() -> (w6787:sgl[])
                n2128 = Greater?(x=w6778, y=w6777) -> (0:w6796:bool)
                n2129 = Build Array (concatenate)(w6787, w6777) -> (w6788:sgl[])
                n2130 = Compound Arithmetic op=AND(w6796, w6789) -> (→"Focus index recovery active":bool)
                n2131 = local write "FI low limit array"(w6788) -> ()
              }
              frame #22 {
                n2132 = local read "Auto Align"() -> (w6839:bool)
                n2133 = local read "Auto Focus"() -> (w6835:bool)
                n2134 = local read "Auto Stig"() -> (w6838:bool)
                n2135 = local read "Focus Index tiled"() -> (w6836:sgl[][])
                n2136 = local read "Focus Index array tiled"() -> (w6837:sgl[][][][])
                n2137 = for {
                  tunnel: w6836 -> [w6847] mode=indexing
                  tunnel: [w6846] -> w6834 mode=indexing
                  tunnel: [w6845] -> w6833 mode=indexing
                  tunnel: w6835 -> [w6844]
                  tunnel: w6837 -> [w6843] mode=indexing
                  tunnel: w6838 -> [w6842]
                  tunnel: w6839 -> [w6841]
                  i -> [w6840]
                  n2138 = for {
                    tunnel: w6847 -> [w6857] mode=indexing
                    tunnel: [w6856] -> w6846 mode=indexing
                    tunnel: [w6855] -> w6845 mode=indexing
                    tunnel: w6844 -> [w6852]
                    tunnel: w6843 -> [w6854] mode=indexing
                    tunnel: w6842 -> [w6851]
                    tunnel: w6841 -> [w6850]
                    tunnel: w6840 -> [w6849]
                    i -> [w6848]
                    n2139 = Compound Arithmetic op=OR(w6852, w6851, w6850) -> (w6853:bool)
                    n2140 = case shown="True" w6853 {
                      tunnel: w6857 -> [_ w6883]
                      tunnel: w6854 -> [_ w6882]
                      tunnel: [w6859 w6881] -> w6856
                      tunnel: [w6858 w6880] -> w6855
                      tunnel: w6852 -> [_ w6877]
                      tunnel: w6851 -> [_ w6875]
                      tunnel: w6850 -> [_ w6873]
                      tunnel: w6849 -> [_ w6865]
                      tunnel: w6848 -> [_ w6864]
                      frame False {
                        n2141 = local read "FI grid array"() -> (w6858:sgl[][][])
                        n2142 = local read "FI array"() -> (w6859:sgl[])
                      }
                      frame True {
                        w6879 = u8 1 ("AF Count")
                        n2143 = local read "AF Count"() -> (w6862:u8)
                        n2144 = local read "AS Count"() -> (w6860:u8)
                        n2145 = local read "AA Count"() -> (w6861:u8)
                        n2146 = local read "FI array tiled"() -> (w6868:sgl[][][])
                        n2147 = local read "FI grid array tiled"() -> (w6866:sgl[][][][][])
                        n2148 = Index Array(array=w6868, index (dim 0)=w6865, index (dim 1)=w6864) -> (element=w6867:sgl[])  [unwired: 1 in]
                        n2149 = Index Array(array=w6866, index (dim 0)=w6865, index (dim 1)=w6864) -> (element=w6863:sgl[][][])  [unwired: 3 in]
                        n2150 = Equal?(x=w6862, y=w6879) -> (x = y?=w6878:bool)
                        n2151 = Equal?(x=w6860, y=w6879) -> (x = y?=w6876:bool)
                        n2152 = Equal?(x=w6861, y=w6879) -> (x = y?=w6874:bool)
                        n2153 = And(x=w6877, y=w6878) -> (x .and. y?=w6872:bool)
                        n2154 = And(x=w6875, y=w6876) -> (x .and. y?=w6871:bool)
                        n2155 = And(x=w6873, y=w6874) -> (x .and. y?=w6870:bool)
                        n2156 = Compound Arithmetic op=OR(w6872, w6871, w6870) -> (w6869:bool)
                        n2157 = case shown="False" w6869 {
